vi "DQMH Request UI Display (Cloneable).vi"(7 "Module Disk Path":path, 8 "error in (no error)":errorcluster, 9 "Display Scenario":T1, 10 "Module ID":i32=-1, 11 "Application reference":refnum<vi>) -> (0 "error out":errorcluster, 3 "Accept?":bool)   [LabVIEW 2020, in "hse-dqmh-dynamicrequesters.lvlib"]
doc: "Calls the \"Request UI Display\" request VI of the module in <b>Path to module directory</b>. Hands over the <b>Module ID</b> and the <b>Display Scenario</b>.\n\n____\nHAMPEL SOFTWARE ENGINEERING v3.8.0 (2023-12-18 14:41)"
uses:
  hse-dqmh-dynamicrequesters.lvlib
  Controls/Module Display Scenarios.ctl
  hse-dqmh.lvlib
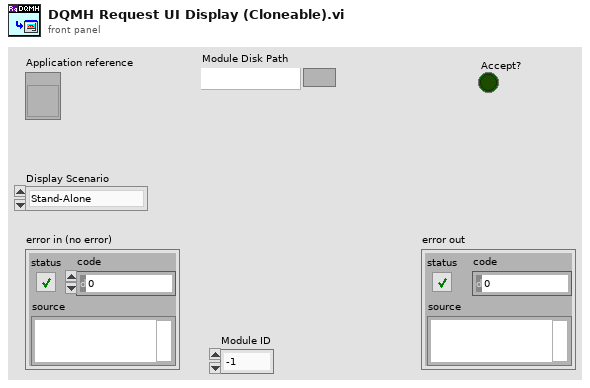
[diagram p1: front panel]
types:
  T1 = typedef "hse-dqmh.lvlib/Module Display Scenarios.ctl" = enum16{"Stand-Alone", "Managed"}
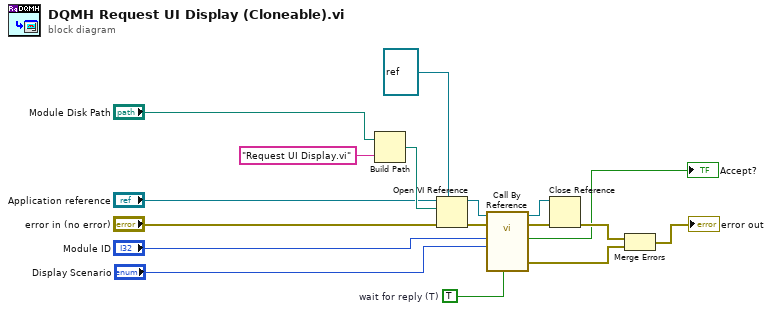
[diagram p0: block diagram]
diagram:
  w2 = TRUE  # wait for reply (T)
  n1 = Build Path(base path="Module Disk Path", name or relative path="Request UI Display.vi") -> (appended path=w15:path)
  n2 = Open VI Reference(type specifier VI Refnum (for type only)=refnum<vi> refnum, application reference (local)="Application reference", vi path=w15, error in (no error)="error in (no error)") -> (vi reference=w17:refnum<vi>, error out=w12:errorcluster)  [unwired: 2 in]
  n3 = call-by-ref "?"(reference=w17, error in=w12, "wait for reply (T)"=w2, "Scenario"="Display Scenario", "Module ID"="Module ID") -> (reference out=w9:refnum<vi>, error out=w13:errorcluster, 0:"error out"=w14:errorcluster, "Accept?"=→"Accept?":bool)  [unwired: 7 in]
  n4 = Close Reference(reference=w9, error in (no error)=w13) -> (error out=w10:errorcluster)
  n5 = Merge Errors(w10, w14) -> (→"error out":errorcluster)
